vi "get_spill_id.vi"() -> (0 "status":bool, 3 "spill_id":i32)   [LabVIEW 2019]
panel:
  out "text":string
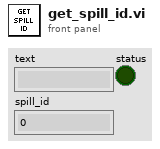
[diagram p1: front panel]
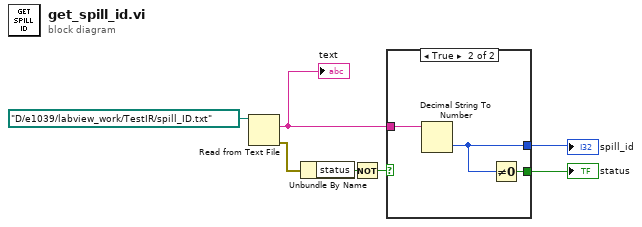
[diagram p0: block diagram]
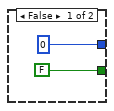
[diagram p2: hidden frame]
diagram:
  n1 = Read from Text File(file (use dialog)=path "D:/e1039/labview_work/TestIR/spill_ID.txt") -> (text=w6:string, error out=w5:errorcluster)  [unwired: 3 in, 2 out]
  "text" <- w6
  n2 = Unbundle By Name(w5) -> ("status"=w4:bool)
  n3 = Not(x=w4) -> (.not. x?=w3:bool)
  n4 = case shown="True" w3 {
    tunnel: w6 -> [_ w12]
    tunnel: [0 w11] -> w2
    tunnel: [FALSE w10] -> w1
    frame False {
    }
    frame True {
      n5 = Decimal String To Number(string=w12) -> (number=w11:i32)  [unwired: 2 in, 1 out]
      n6 = Not Equal To 0?(x=w11) -> (x != 0?=w10:bool)
    }
  }
  "spill_id" <- w2
  "status" <- w1
